vi "Do.vi"(8 "error in (no error)":errorcluster, 10 "Actor in":refnum<class "Actor.lvclass">, 11 "Start measurements Msg":refnum<class "Start measurements Msg.lvclass">) -> (0 "error out":errorcluster, 2 "Actor out":refnum<class "Actor.lvclass">)   [LabVIEW 2015, in "Start measurements Msg.lvclass"]
doc: "This VI delivers the message to the actor by calling the appropriate method(s) on the actor."
uses:
  Start measurements Msg.lvclass
  <vilib>/ActorFramework/Actor/Actor.lvclass
  Mag Lab Measure Controller/Mag Lab Measure Controller.lvclass
  Start measurements Msg.lvclass/Start measurements Msg.ctl
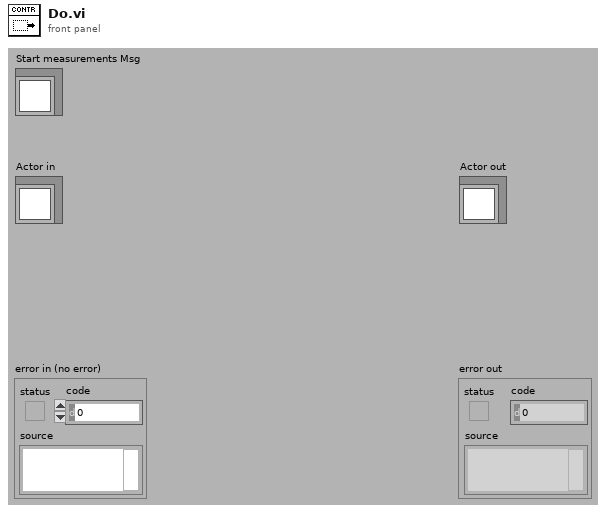
[diagram p1: front panel]
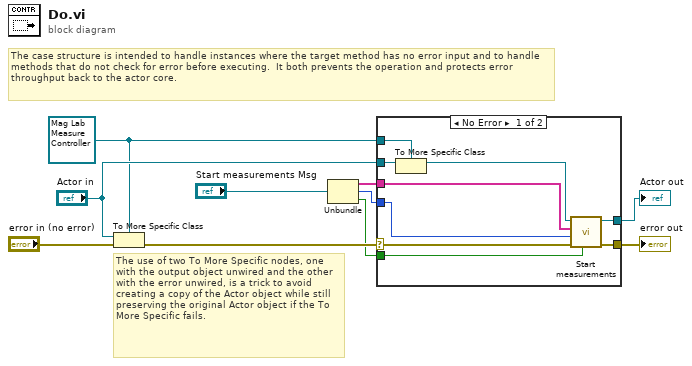
[diagram p0: block diagram]
diagram:
  w4 = refnum<class "Mag Lab Measure Controller.lvclass"> refnum ("Actor in")
  # "The use of two To More Specific nodes, one with the output object unwired and the other with the error unwired, is a trick to avoid creating a copy of the Actor object while still preserving the original Actor object if the To More Specific fails."
  # "The case structure is intended to handle instances where the target method has no error input and to handle methods that do not check for error before executing.  It both prevents the operation and protects error throughput back to the actor core."
  n1 = To More Specific Class(target class=w4, reference="Actor in", error in="error in (no error)") -> (error out=w8:errorcluster)  [unwired: 1 out]
  n2 = Unbundle("Start measurements Msg") -> (w3:string[], w2:i32, w1:bool)
  n3 = case shown="No Error" w8 {
    selector: w8 -> [w17 w21]
    tunnel: [w19 w21] -> w7
    tunnel: [w18 w20] -> w6
    tunnel: "Actor in" -> [w16 w20]
    tunnel: w4 -> [w15 _]
    tunnel: w3 -> [w13 _]
    tunnel: w2 -> [w12 _]
    tunnel: w1 -> [w11 _]
    frame No Error {
      n4 = To More Specific Class(target class=w15, reference=w16) -> (specific class reference=w14:refnum<class "Mag Lab Measure Controller.lvclass">)  [unwired: 1 in, 1 out]
      n5 = call-dynamic "Start measurements.vi"("Syncronize measurements"=w11, "error in (no error)"=w17, "Repeat times"=w12, "Measurements"=w13, "Mag Lab Measure Controller in"=w14) -> ("error out"=w19:errorcluster, "Mag Lab Measure Controller out"=w18:refnum<class "Mag Lab Measure Controller.lvclass">)  [unwired: 5 in]
    }
    frame Error {
      # "If type check fails, pass the original object out again."
    }
  }
  "error out" <- w7
  "Actor out" <- w6
